vi "picoscopePythonAnalyisForCharge.vi"(8 "error in (no error)":errorcluster, 11 "PicoscopeV2 in":refnum<class "PicoscopeV2.lvclass">) -> (0 "error out":errorcluster, 3 "PicoscopeV2 out":refnum<class "PicoscopeV2.lvclass">)   [LabVIEW 2020, in "PicoscopeV2.lvclass"]
uses:
  PicoscopeV2.lvclass
  shared/OnOffTypeDef.ctl
  PicoscopeV2.lvclass/PicoscopeV2.ctl
  shared/CompressAndUpdate(Poly)/CompressAndUpdate(Numeric).vi
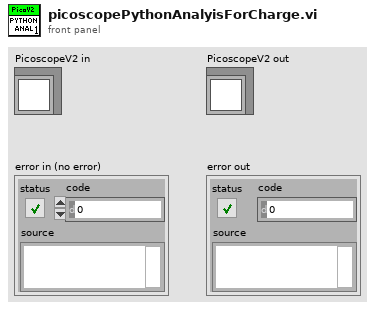
[diagram p1: front panel]
types:
  T1 = typedef "OnOffTypeDef.ctl" = enum16{"off", "on"}
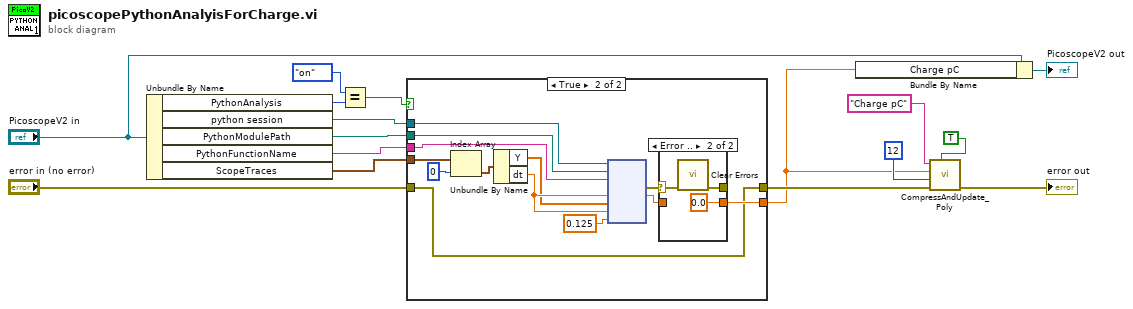
[diagram p0: block diagram]
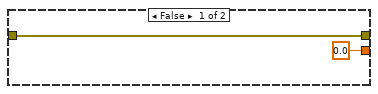
[diagram p2: hidden frame]
diagram:
  n1 = Unbundle By Name("PicoscopeV2 in") -> ("PythonAnalysis"=w1:T1, "python session"=w4:refnum<k35>, "PythonModulePath"=w5:path, "PythonFunctionName"=w6:string, "ScopeTraces"=w7:waveform(dbl)[])
  n2 = Equal?(x=OnOffTypeDef."on", y=w1) -> (x = y?=w3:bool)
  n3 = case shown="True" w3 {
    tunnel: w4 -> [_ w24]
    tunnel: w5 -> [_ w23]
    tunnel: w6 -> [_ w22]
    tunnel: w7 -> [_ w21]
    tunnel: [0.0 ("dt") w20] -> w10
    tunnel: "error in (no error)" -> [w17 w19]
    tunnel: [w17 w19] -> w14
    frame False {
    }
    frame True {
      n4 = Index Array(array=w21, index=0 ("disabled index (col)")) -> (element=w25:waveform(dbl))
      n5 = Unbundle By Name(w25) -> ("Y"=w27:dbl[], "dt"=w29:dbl)
      n6 = node(w24, w23, w22, w29, w27, w29, 0.125 ("Numeric")) -> (w30:errorcluster, w31:dbl)  [unwired: 4 in, 3 out]
      n7 = case shown="Error .." w30 {
        selector: w30 -> [w32 w35]
        tunnel: w31 -> [w33 _]
        tunnel: [w33 0.0 ("dt")] -> w20
        tunnel: [w32 w34] -> _
        frame No Error {
        }
        frame Error {
          n8 = call <vilib>:"Clear Errors.vi"("error in (no error)"=w35) -> ("error out"=w34:errorcluster)  [unwired: 5 in, 1 out]
        }
      }
    }
  }
  n9 = Bundle By Name(cluster="PicoscopeV2 in", "Charge pC"=w10) -> (→"PicoscopeV2 out":refnum<class "PicoscopeV2.lvclass">)
  n10 = call-poly "CompressAndUpdate_Poly.vi"("force CVT update (false)"=TRUE, "error in"=w14, "precision (6)"=i16 12, "Numeric"=w10, "command or variable name"="Charge pC") -> ("error out"=→"error out":errorcluster)  [unwired: 6 in]
